vi "CH_LM Config Range Auto.vi"(0 "Meter Index":i32, 2 "Auto Range (disable)":bool, 5 "error in (no error)":errorcluster, 7 "Timeout / ms (3000)":i32=3000, 8 "Action (query)":bool, 9 "Lock Timeout / ms (1000)":i32=1000) -> (11 "Lock timed out":bool, 14 "Meter Index":i32, 16 "Auto Range":bool, 19 "error out":errorcluster)   [LabVIEW 2012, in "CH_LM.lvlib"]
doc: "This command will set/query enable or disable automatic selection of the meter measurement range.\n\nThe meter will hunt for the best measurement range for the current probe and laser conditions when auto ranging is active. The hunt procedure may require several samples to arrive at the best range. Auto ranging will apply only when a thermopile or optical probe is attached."
uses:
  CH_LM.lvlib
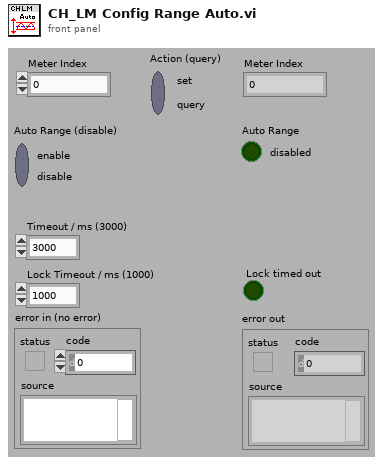
[diagram p1: front panel]
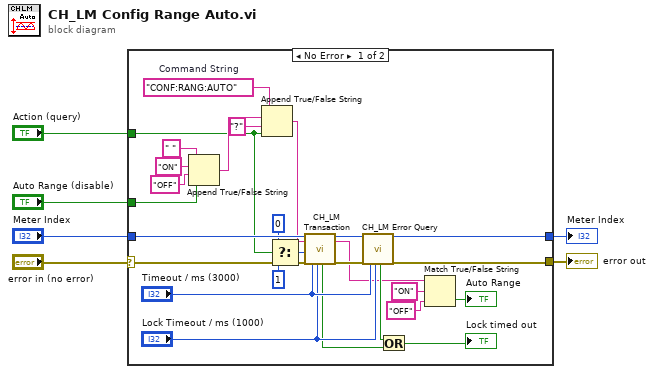
[diagram p0: block diagram]
diagram:
  n1 = case shown="No Error" "error in (no error)" {
    selector: "error in (no error)" -> [w33 w35]
    tunnel: [w31 w35] -> w6
    tunnel: "Meter Index" -> [w32 w34]
    tunnel: [w30 w34] -> w3
    tunnel: "Auto Range (disable)" -> [w22 _]
    tunnel: "Action (query)" -> [w14 _]
    frame No Error {
      w19 = "CONF:RANG:AUTO"  # Command String
      n2 = Append True/False String(1:w22, 2:"OFF" ("false string"), 3:"ON" ("true string"), 4:" " ("string (\"\")")) -> (0:w16:string)
      n3 = Append True/False String(1:w14, 2:"?", 3:w16, 4:w19) -> (0:w15:string)
      n4 = Select(t=0, s=w14, f=1) -> (s? t:f=w12:i32)
      n5 = call "CH_LM Transaction.vi"("Meter Index"=w32, "Command String"=w15, "NofStrings (-1:all)"=w12, "error in (no error)"=w33, "Timeout / ms (3000)"="Timeout / ms (3000)", "Lock Timeout / ms (1000)"="Lock Timeout / ms (1000)") -> ("Lock timed out"=w24:bool, "Meter Index"=w27:i32, "Response"=w9:string, "error out"=w26:errorcluster)  [unwired: 10 out]
      n6 = call "CH_LM Error Query.vi"("Meter Index"=w27, "error in (no error)"=w26, "Timeout / ms (3000)"="Timeout / ms (3000)", "Lock Timeout / ms (1000)"="Lock Timeout / ms (1000)") -> ("Lock timed out"=w25:bool, "Meter Index"=w30:i32, "error out"=w31:errorcluster)  [unwired: 13 out]
      n7 = Or(x=w25, y=w24) -> (x .or. y?=→"Lock timed out":bool)
      n8 = Match True/False String(2:"OFF" ("false string"), 3:"ON" ("true string"), 4:w9) -> (0:→"Auto Range":bool)  [unwired: 1 out]
    }
    frame Error {
    }
  }
  "error out" <- w6
  "Meter Index" <- w3
